vi "Global_archivobasedatos.vi"() -> ()   [LabVIEW 2020]
doc: "Variable Global que contiene el path del archivo .udl necesario para el funcionamiento de las funciones del módulo de conectividad y bases de datos."
panel:
  in  "Path":path=path "D:/Universidad/8voSemestre/Labview2/Proyecto Final/objetos3d.udl"
  # "Especificar el path del archivo .udl de la base de datos que se quiere conectar"
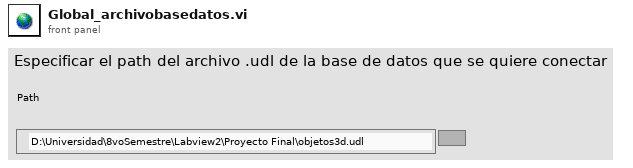
[diagram p1: front panel]
diagram:
